vi "Teleop Drivetrain Control.vi"(8 "Manip Button Cluster":T1, 9 "D-Pad":T2, 10 "Driver Button Cluster":T1, 11 "Axes":T3) -> ()   [LabVIEW 2015]
uses:
  Common Code/Gamepads/Axes Cluster.ctl
  Common Code/Gamepads/Button Cluster.ctl
  Common Code/Gamepads/D-Pad.ctl
  Common Code/Drivetrain Modes.ctl
  Common Code/Catapult/Shoot Mode.ctl
  Common Code/Change Detect.vi
  Common Code/Change Detect Boolean.vi
  Robot Global Data.vi
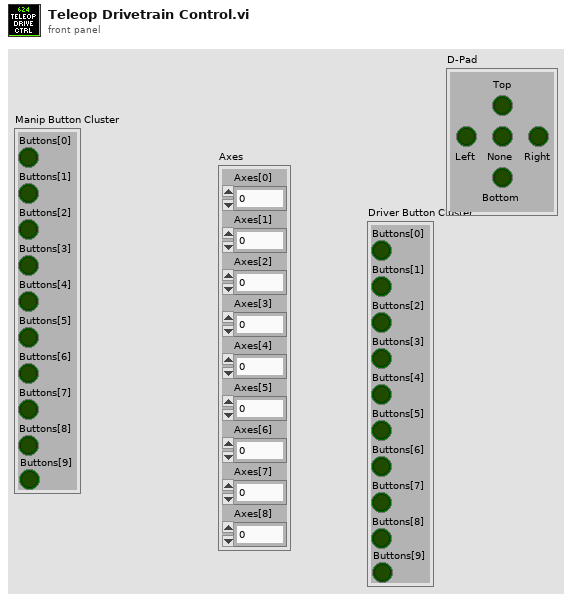
[diagram p1: front panel]
types:
  T1 = typedef "Button Cluster.ctl" = cluster{"Buttons[0]":bool, "Buttons[1]":bool, "Buttons[2]":bool, "Buttons[3]":bool, "Buttons[4]":bool, "Buttons[5]":bool, "Buttons[6]":bool, "Buttons[7]":bool, "Buttons[8]":bool, "Buttons[9]":bool}
  T2 = typedef "D-Pad.ctl" = cluster{"Top":bool, "Bottom":bool, "None":bool, "Right":bool, "Left":bool}
  T3 = typedef "Axes Cluster.ctl" = cluster{"Axes[0]":dbl, "Axes[1]":dbl, "Axes[2]":dbl, "Axes[3]":dbl, "Axes[4]":dbl, "Axes[5]":dbl, "Axes[6]":dbl, "Axes[7]":dbl, "Axes[8]":dbl}
  T4 = typedef "Shoot Mode.ctl" = enum16{"Outer", "Batter"}
  T5 = typedef "Drivetrain Modes.ctl" = enum16{"Gyro Steer", "Climb", "Manual", "Goal Vision Targeting", "PID Distance Drive", "Hybrid"}
  T6 = typedef "Catapult Command Cluster.ctl" = cluster{"States":T7, "Mode":T8, "Override IR":bool, "Shoot Mode":T4, "Ball Loaded?":bool, "High Pressure?":bool, "Shoot?":bool}
  T7 = typedef "Catapult Auto Commands.ctl" = enum16{"Idle", "Warmup", "Shoot"}
  T8 = typedef "Shoot Modes Enum.ctl" = enum16{"Auto"}
  T9 = typedef "Drivetrain Commands.ctl" = cluster{"Y Power":dbl, "Turn Power":dbl, "Modes":T5, "Heading Target":dbl, "X Max Speed":dbl, "Y Max Speed":dbl, "X Min Speed":dbl, "Y Min Speed":dbl, "Y Target":dbl, "Max Accel":dbl, "Max Velocity":dbl, "Pivot Speed":dbl}
  T10 = typedef "Climb Command Cluster.ctl" = cluster{"Climb Mode":T11, "Hold?":bool, "Manual State":T12}
  T11 = typedef "Climb Mode.ctl" = enum16{"Auto", "Semi-Auto", "Manual"}
  T12 = typedef "Climb Manual State.ctl" = cluster{"Release":bool, " PTO Engage":bool, "Extend":bool}
  T13 = typedef "Dashboard Control Data.ctl" = cluster{"Shooter Presets":T14, "Encoder Control":T16, "Steer PID output":cluster{"output high":dbl, "output low":dbl}, " Steer PID gains":cluster{"proportional gain (Kc)":dbl, "integral time (Ti, min)":dbl, "derivative time (Td, min)":dbl}, "Drivetrain Settings":T17, "Vision Packet":T18, "Dashboard Drivetrain Command":T19, "Info/Command Cluster":T21, "Ball Vision Packet":T22, "Intake Presets":T24, "Intake Encoder Control":T26, "Climb Presets":T27, "Goal Output Range":cluster{"output high":dbl, "output low":dbl}, "Enabled Systems":T28, "Auton Presets":T29, "Pressure M":dbl, "Pressure B":dbl, "Vision Timeout":dbl, "Auto-Shift":T30, "Catapult Setpoints":T31}
  T14 = typedef "Shooter Presets.ctl" = cluster{"Batter Shot":T15, "Deep Middle":T15, "Manual Shot":T15, "Left Ticks Per Rotation":dbl, "Right Ticks Per Rotation":dbl, "Low Bar Shot":T15, "Shooter RPM Tolerance":dbl, "Trigger Power":dbl, "Fire from Load Delay":i32, "Max Angle":dbl, "Min Angle":dbl, "Angle PID gains":cluster{"P":dbl, "I":dbl, "D":dbl}, "Angle Output":cluster{"output high":dbl, "output low":dbl}, "Shooter Angle Tolerance":dbl, "Vision Shoot x^2":dbl, "Vision Shoot x":dbl, "Feed Forward Max Accel":dbl, "Feed Forward Kv":dbl, "Backwards Trigger":dbl, "Shot Finish Delay (ms)":dbl, "Angle Max Current":dbl, "Angle Current Trip Time":dbl, "Intake Angle":dbl, "Vision Shoot c":dbl, "Reset?":bool, "Button Release Delay":dbl, "Angle Pot x":dbl, "Angle Pot c":dbl, "Ignore Angle?":bool, "Max RPM":dbl, "Safty Frist Angle":dbl, "Intake Danger Height":dbl, "Angle Pot B":i32, "Angle Pot M":dbl, "FF Finish RPM":dbl, "RPM PID Right":cluster{"P":dbl, "I":dbl, "D":dbl, "FF":dbl}, "RPM PID Left":cluster{"P":dbl, "I":dbl, "D":dbl, "FF":dbl}, "Backwards RPM":dbl, "Vision RPM":dbl, "Run Wheels Backward Delay":u32, "Cleat Shot":T15, "Vision Far RPM":dbl, "Vision Far Distance":dbl, "Vision Far Angle":dbl}
  T15 = typedef "Shot Presets.ctl" = cluster{"L":dbl, "R":dbl, "A":dbl}
  T16 = typedef "Encoder Control.ctl" = cluster{"Right Tick Constant":dbl, "Left Tick Constant":dbl, "Reset?":bool, "Y Dist":cluster{"PID gains":cluster{"proportional gain (Kc)":dbl, "integral time (Ti, min)":dbl, "derivative time (Td, min)":dbl}}, "Y Stop Thresh":dbl, "Y Stop Speed":dbl}
  T17 = typedef "Drivetrain Settings.ctl" = cluster{"Gyro Tolerance":dbl, "Throttle Ramp (ms)":dbl, "Kv":dbl, "Ka":dbl, "Feed Forward P":dbl, "Feed Forward D":dbl, "Goal Vision PID gains":cluster{"proportional gain (Kc)":dbl, "integral time (Ti, min)":dbl, "derivative time (Td, min)":dbl}, "Goal Detection Window":dbl, "Creep Rate":dbl, "Vision Throttle Threshold":dbl, "Min Turn Output":dbl, "Left Batter Angle":dbl, "Right Batter Angle":dbl}
  T18 = typedef "Goal Vision Packet.ctl" = cluster{"Distance":dbl, "Center X":dbl, "Center Y":dbl, "Found Target?":bool, "Robot Center":dbl, "Angle":dbl}
  T19 = typedef "Dashboard Drivetrain Command.ctl" = cluster{"Drivetrain Vision":T20}
  T20 = typedef "Drivetrain Vision.ctl" = cluster{"Goal Window":dbl, "Ball Window":dbl}
  T21 = typedef "Ball Tracking Command Cluster.ctl" = cluster{"Distance to Ball":dbl, "Desired Angle":dbl, "Command":enum16{"Turn to Ball", "Turn to Angle", "Get Distance"}, "Pixels from Center":dbl}
  T22 = typedef "Ball Vision Packet.ctl" = cluster{"Ball Detected?":bool, "Distance to Ball":dbl, "Desired Angle":dbl, "Pixels from Center":dbl, "Tracking mode":T23}
  T23 = typedef "Tracking Mode.ctl" = enum16{"Turn to Ball", "Turn to Angle"}
  T24 = typedef "Intake Presets.ctl" = cluster{"Intake Speed":dbl, "Outake Speed":dbl, "Low Height":dbl, "Half Height":dbl, "High Idle Height":dbl, "Angle Speed":dbl, "Angle Tolerance":dbl, "Encoder Scale":dbl, "Load Height":dbl, "Output Range":T25, "Rotation Power Max/Min":dbl, "MaxCurrent":dbl, "Intake Trip Time":dbl, "Idle Height":dbl, "Max Height":dbl, "Reset Encoders?":bool, "PID gains":cluster{"proportional gain (Kc)":dbl, "integral time (Ti, min)":dbl, "derivative time (Td, min)":dbl}, "Intake Stop Delay":u32, "Settle Time":dbl, "Settle Wait Time":dbl, "Pull Up Delay":dbl}
  T25 = typedef "Drivetrain Output Range.ctl" = cluster{"output high":dbl, "output low":dbl}
  T26 = typedef "IntakeEcoderControl.ctl" = cluster{"Arm Tick Constant":dbl, "Reset?":bool, "Y Dist":cluster{"PID gains":cluster{"proportional gain (Kc)":dbl, "integral time (Ti, min)":dbl, "derivative time (Td, min)":dbl}}, "Y Stop Thresh":dbl, "Y Stop Speed":dbl}
  T27 = typedef "Climb Presets.ctl" = cluster{"Pull Power":dbl, "Extend Power":dbl}
  T28 = typedef "Enabled Systems.ctl" = cluster{"Shoot":bool, "Intake":bool, "DT":bool, "Gyro":bool, "100ms":bool, "US":bool}
  T29 = typedef "Autonomous Presets.ctl" = cluster{"Pitch Limit":dbl, "Roll Limit":dbl, "Start Position":dbl, "Cross Position":dbl}
  T30 = typedef "Auto Shift Cluster.ctl" = cluster{"Delay":dbl, "Speed Thresh":dbl, "Upshift Accel":dbl, "Upshift Throttle":dbl, "Upshift Throttle Accel":dbl, "Downshift Throttle":dbl, "Downshift Throttle Accel":dbl, "Pressure Threshold":dbl}
  T31 = typedef "Catapult Presets.ctl" = cluster{"Intake Danger Height":dbl, "Ball Security Delay ":dbl, "High PSI Minimum":dbl, "Shot Finish Delay":dbl, "Low PSI Minimum":dbl}
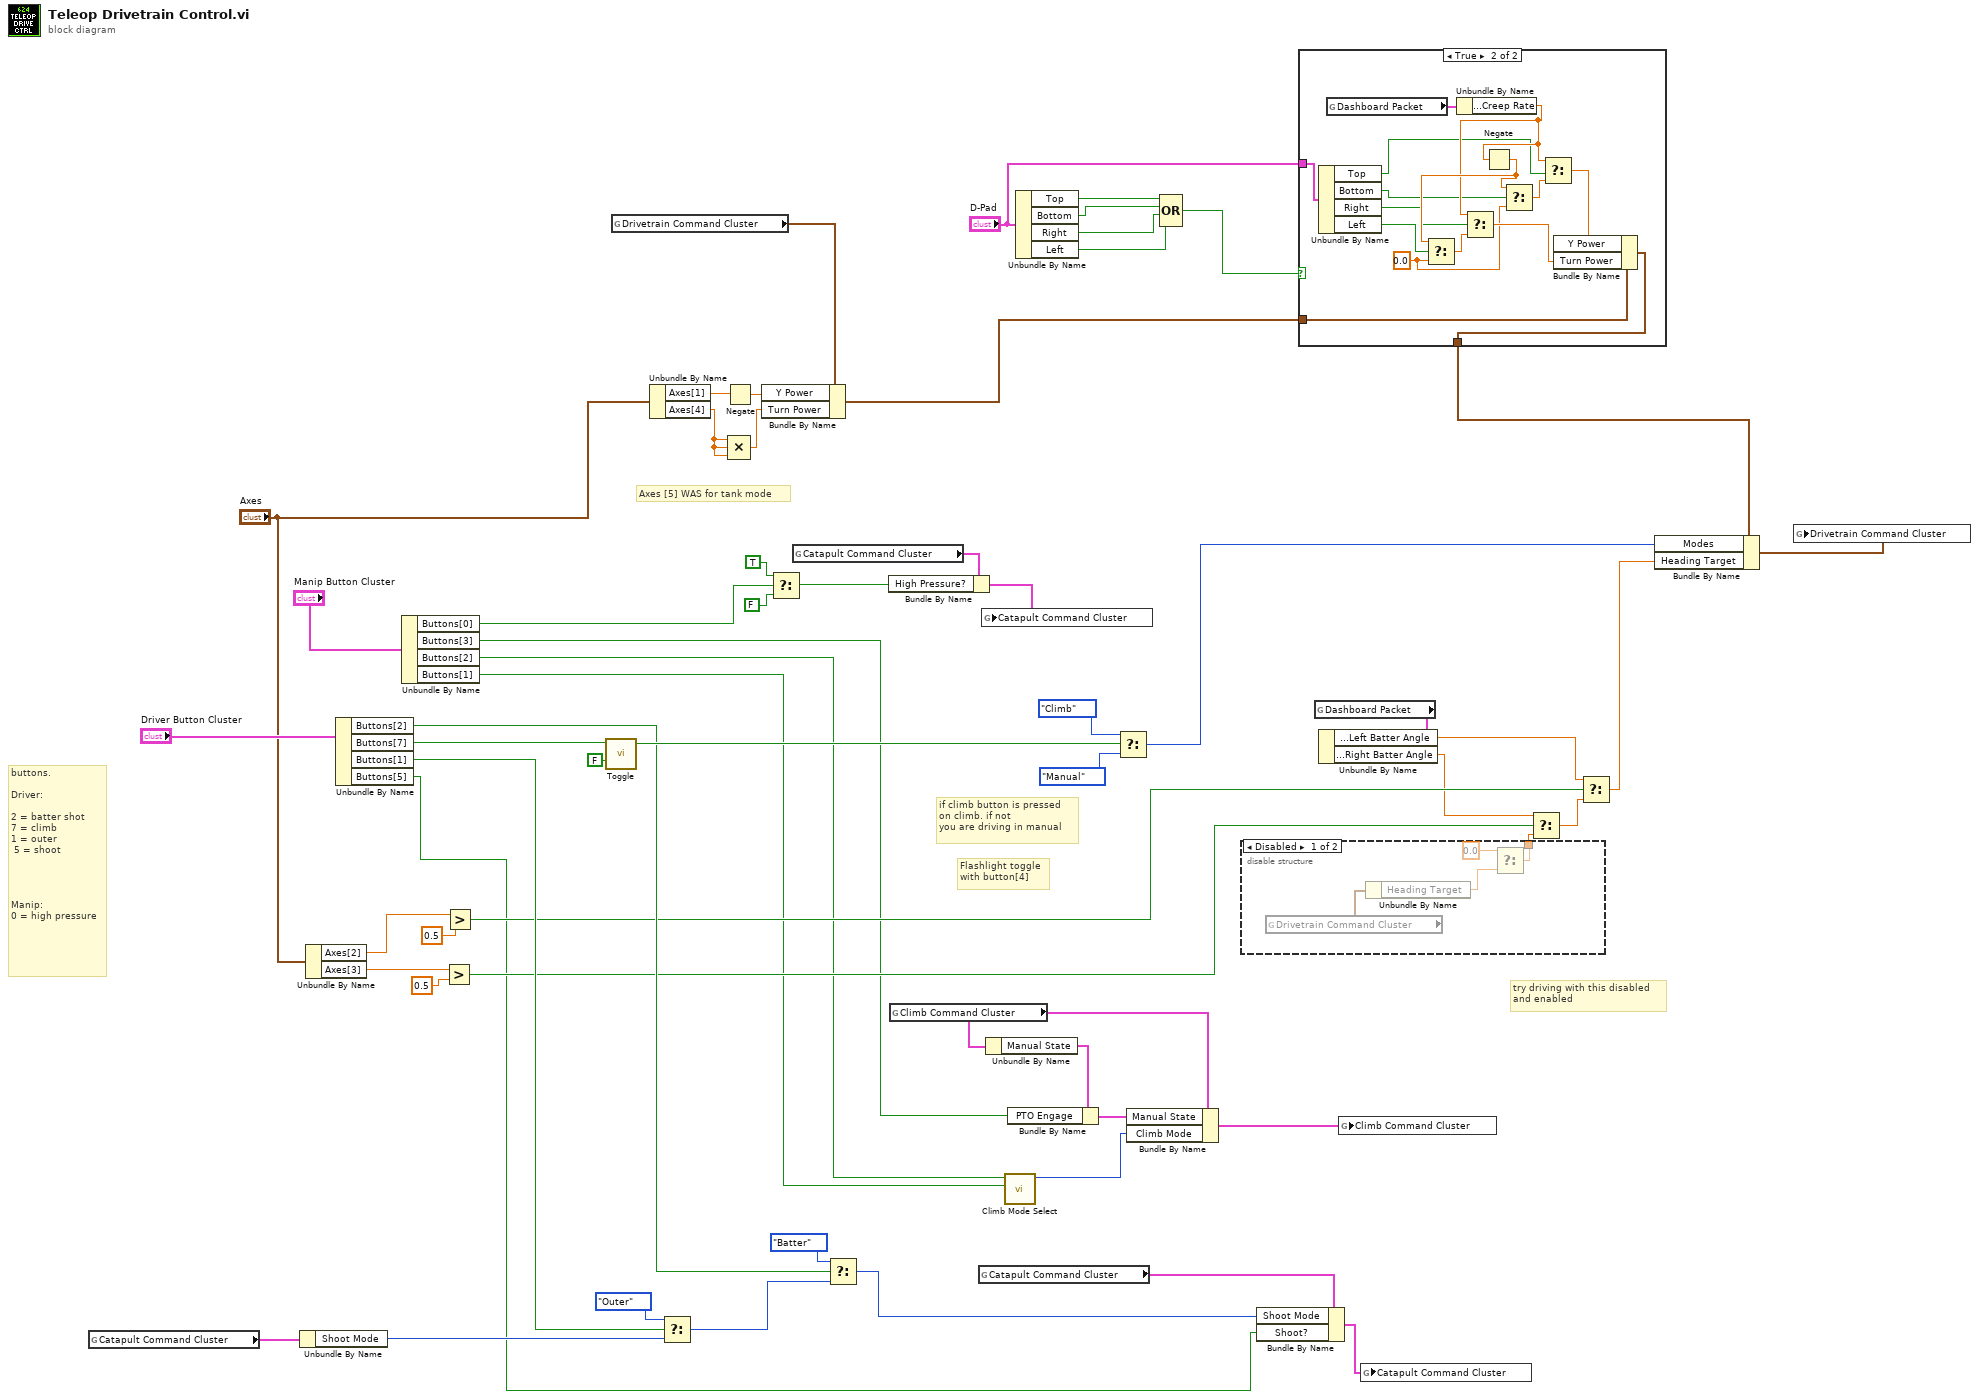
[diagram p0: block diagram]
diagram:
  # "try driving with this disabled \nand enabled"
  # "if climb button is pressed\non climb. if not\nyou are driving in manual"
  # "buttons.\n\nDriver:\n\n2 = batter shot \n7 = climb\n1 = outer \n 5 = shoot \n\n\n\n\nManip:\n0 = high pressure"
  # "Axes [5] WAS for tank mode"
  # "Flashlight toggle\nwith button[4]"
  n1 = global read "Robot Global Data.vi" "Catapult Command Cluster"() -> (w27:T6)
  n2 = Unbundle By Name(w27) -> ("Shoot Mode"=w26:T4)
  n3 = Unbundle By Name("Axes") -> ("Axes[2]"=w24:dbl, "Axes[3]"=w22:dbl)
  n4 = Unbundle By Name("Driver Button Cluster") -> ("Buttons[2]"=w39:bool, "Buttons[7]"=w56:bool, "Buttons[1]"=w37:bool, "Buttons[5]"=w1:bool)
  n5 = Unbundle By Name("Manip Button Cluster") -> ("Buttons[0]"=w33:bool, "Buttons[3]"=w6:bool, "Buttons[2]"=w4:bool, "Buttons[1]"=w5:bool)
  n6 = Greater?(x=w22, y=0.5) -> (0:w18:bool)
  n7 = Greater?(x=w24, y=0.5) -> (0:w19:bool)
  n8 = call "Toggle.vi"("Initial Value"=FALSE, "In"=w56) -> ("Toggled"=w43:bool)  [unwired: 9 in]
  n9 = global read "Robot Global Data.vi" "Drivetrain Command Cluster"() -> (w44:T9)
  n10 = Unbundle By Name("Axes") -> ("Axes[1]"=w45:dbl, "Axes[4]"=w42:dbl)
  n11 = Select(t=Shoot_Mode."Outer" ("Shoot Mode"), s=w37, f=w26) -> (s? t:f=w25:T4)
  n12 = Negate(x=w45) -> (-x=w46:dbl)
  n13 = Compound Arithmetic op=MULTIPLY(w42, w42, w42) -> (w7:dbl)
  n14 = Bundle By Name(cluster=w44, "Y Power"=w46, "Turn Power"=w7) -> (w53:T9)
  n15 = Select(t=TRUE, s=w33, f=FALSE) -> (s? t:f=w28:bool)
  n16 = global read "Robot Global Data.vi" "Catapult Command Cluster"() -> (w30:T6)
  n17 = Select(t=Shoot_Mode."Batter" ("Shoot Mode"), s=w39, f=w25) -> (s? t:f=w2:T4)
  n18 = Bundle By Name(cluster=w30, "High Pressure?"=w28) -> (w29:T6)
  n19 = global read "Robot Global Data.vi" "Climb Command Cluster"() -> (w13:T10)
  n20 = global read "Robot Global Data.vi" "Catapult Command Cluster"() -> (w35:T6)
  n21 = global write "Robot Global Data.vi" "Catapult Command Cluster"(w29) -> ()
  n22 = Unbundle By Name(w13) -> ("Manual State"=w17:T12)
  n23 = call "Climb Mode Select.vi"("Set To Manual?"=w5, "Set To Auto?"=w4) -> ("Mode"=w14:T11)  [unwired: 9 in]
  n24 = Bundle By Name(cluster=w17, "PTO Engage"=w6) -> (w15:T12)
  n25 = Unbundle By Name("D-Pad") -> ("Top"=w52:bool, "Bottom"=w51:bool, "Right"=w50:bool, "Left"=w49:bool)
  n26 = Select(t=Drivetrain_Modes."Climb" ("s? t:f"), s=w43, f=Drivetrain_Modes."Manual") -> (s? t:f=w3:T5)
  n27 = Bundle By Name(cluster=w13, "Manual State"=w15, "Climb Mode"=w14) -> (w16:T10)
  n28 = Compound Arithmetic op=OR(w52, w51, w50, w49) -> (w47:bool)
  n29 = disable-structure shown="Disabled" {
    disable-tunnel: [w62 _] -> w9
    frame Disabled {
      n30 = global read "Robot Global Data.vi" "Drivetrain Command Cluster"() -> (w64:T9)
      n31 = Unbundle By Name(w64) -> ("Heading Target"=w63:dbl)
      n32 = Select(t=0.0, f=w63) -> (s? t:f=w62:dbl)  [unwired: 1 in]
    }
    frame Enabled {
    }
  }
  n33 = Bundle By Name(cluster=w35, "Shoot Mode"=w2, "Shoot?"=w1) -> (w34:T6)
  n34 = case shown="True" w47 {
    tunnel: w53 -> [w65 w79]
    tunnel: [w65 w80] -> w54
    tunnel: "D-Pad" -> [_ w67]
    frame False {
    }
    frame True {
      w66 = 0.0 ("f")
      n35 = Unbundle By Name(w67) -> ("Top"=w71:bool, "Bottom"=w70:bool, "Right"=w69:bool, "Left"=w68:bool)
      n36 = global read "Robot Global Data.vi" "Dashboard Packet"() -> (w74:T13)
      n37 = Unbundle By Name(w74) -> ("Drivetrain Settings.Creep Rate"=w75:dbl)
      n38 = Negate(x=w75) -> (-x=w76:dbl)
      n39 = Select(t=w76, s=w68, f=w66) -> (s? t:f=w72:dbl)
      n40 = Select(t=w75, s=w69, f=w72) -> (s? t:f=w73:dbl)
      n41 = Select(t=w76, s=w70, f=w66) -> (s? t:f=w77:dbl)
      n42 = Select(t=w75, s=w71, f=w77) -> (s? t:f=w78:dbl)
      n43 = Bundle By Name(cluster=w79, "Y Power"=w78, "Turn Power"=w73) -> (w80:T9)
    }
  }
  n44 = global read "Robot Global Data.vi" "Dashboard Packet"() -> (w12:T13)
  n45 = Unbundle By Name(w12) -> ("Drivetrain Settings.Left Batter Angle"=w11:dbl, "Drivetrain Settings.Right Batter Angle"=w8:dbl)
  n46 = global write "Robot Global Data.vi" "Climb Command Cluster"(w16) -> ()
  n47 = global write "Robot Global Data.vi" "Catapult Command Cluster"(w34) -> ()
  n48 = Select(t=w8, s=w18, f=w9) -> (s? t:f=w10:dbl)
  n49 = Select(t=w11, s=w19, f=w10) -> (s? t:f=w41:dbl)
  n50 = Bundle By Name(cluster=w54, "Modes"=w3, "Heading Target"=w41) -> (w60:T9)
  n51 = global write "Robot Global Data.vi" "Drivetrain Command Cluster"(w60) -> ()
